vi "tip data FFT.vi"() -> ()   [LabVIEW 2016]
uses:
  <vilib>/Analysis/4window.llb/windowTd.ctl
  <userlib>/_OpenG.lib/array/array.llb/Sort 1D Array (DBL)__ogtk.vi
  <userlib>/_OpenG.lib/array/array.llb/Reorder 1D Array2 (DBL)__ogtk.vi
  <vilib>/measure/maresamp.llb/Resample Pair of Arrays (single shot).vi
  <vilib>/measure/maspectr.llb/FFT Power Spectrum and PSD for 1 Chan.vi
  <vilib>/measure/NI_MAPro.lvlib
  <vilib>/Analysis/NI_AALPro.lvlib
panel:
  in  "window":T1=3 items=["Rectangle"=0, "Hanning"=1, "Hamming"=2, "Blackman-Harris"=3, "Exact Blackman"=4, "Blackman"=5, "Flat Top"=6, "4 Term B-Harris "=7, "7 Term B-Harris"=8, "Low Sidelobe"=9, "Blackman Nuttall"=11, "Triangle"=30, "Bartlett-Hanning"=31, "Bohman"=32, "Parzen"=33, "Welch"=34, "Kaiser"=60, "Dolph-Chebyshev"=61, "Gaussian"=62]
  in  "t0":dbl=1.15 format="%.2p"
  in  "dt":dbl=1e-05 format="%.2p"
  out "Resampled data":waveform(dbl)(graph)={"t0"=timestamp(1.15 s since 1904-01-01), "dt"=1e-05, "Y"=[]}
  out "FFT (1/um)":cluster{"f0":dbl, "df":dbl, "magnitude":dbl[]}(graph)={"f0"=0.0, "df"=2.940052332931526, "magnitude"=[]}
  out "flattened superlattice":cluster{dbl[], dbl[]}(graph)
  in  "flatten superlattice angle":dbl=-34.65 format="%#_13g"
  in  "superlattice":cluster{dbl[], dbl[]}(graph)
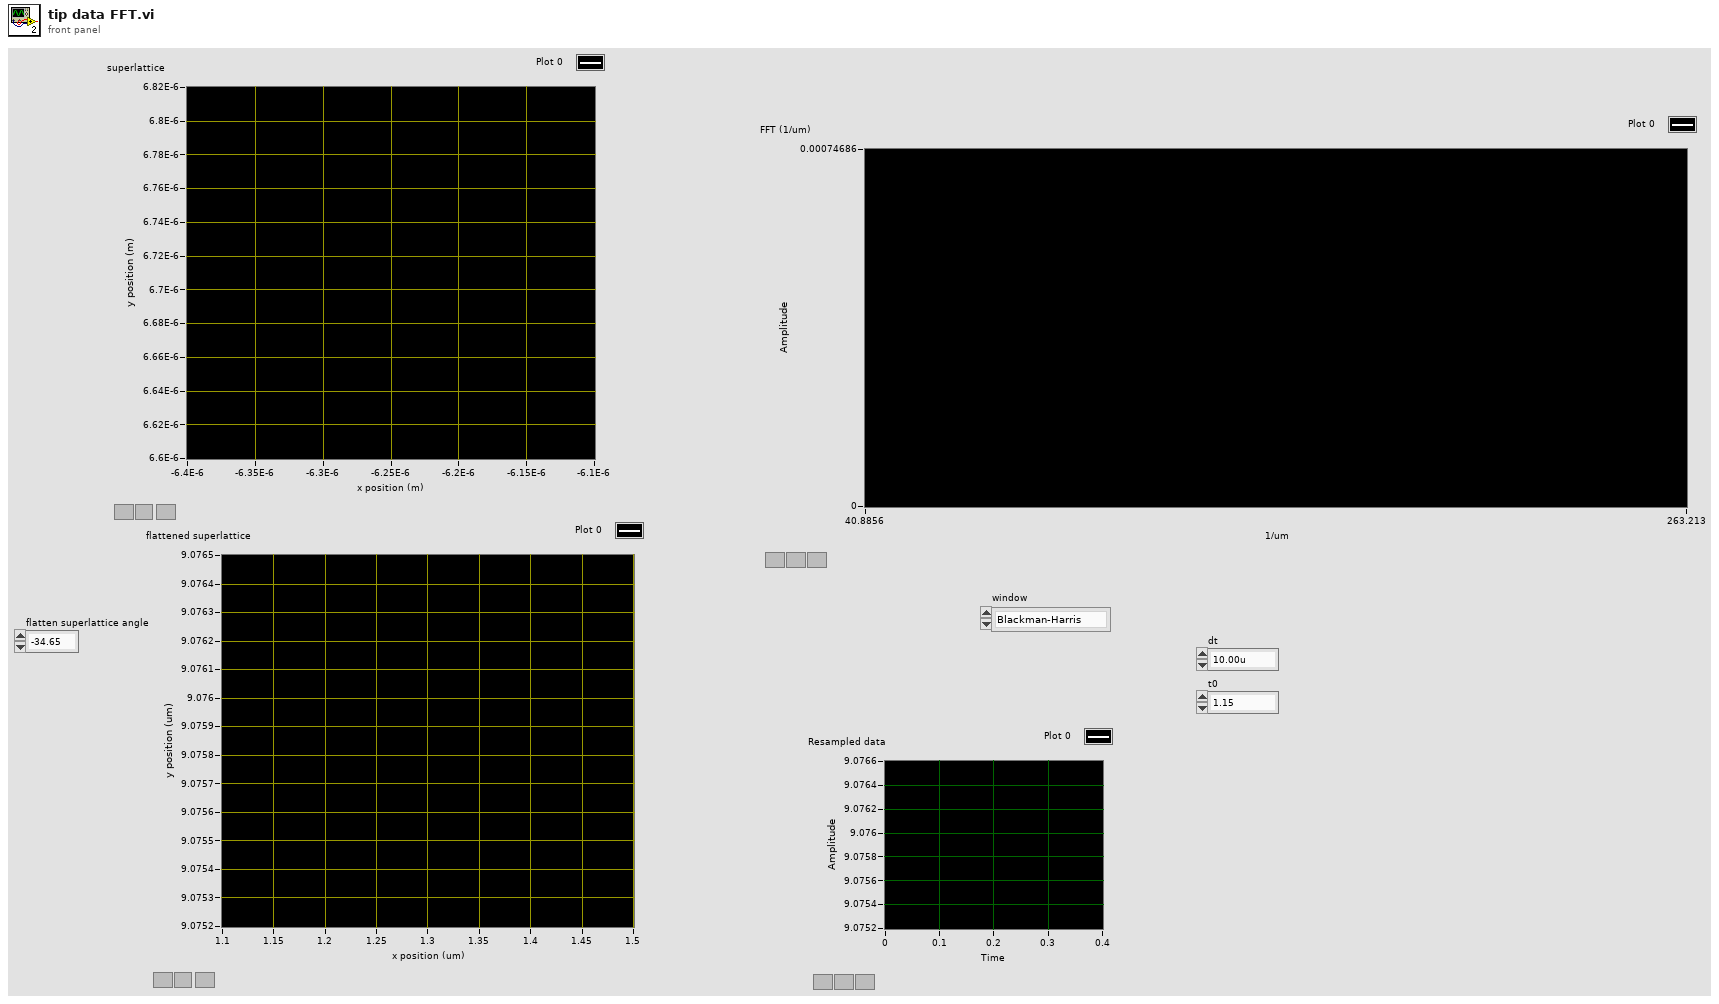
[diagram p1: front panel]
types:
  T1 = typedef "NI_AALPro.lvlib/windowTd.ctl" = u32
  T2 = cluster{"Sorted Array out":dbl[], "reordered array":dbl[]}
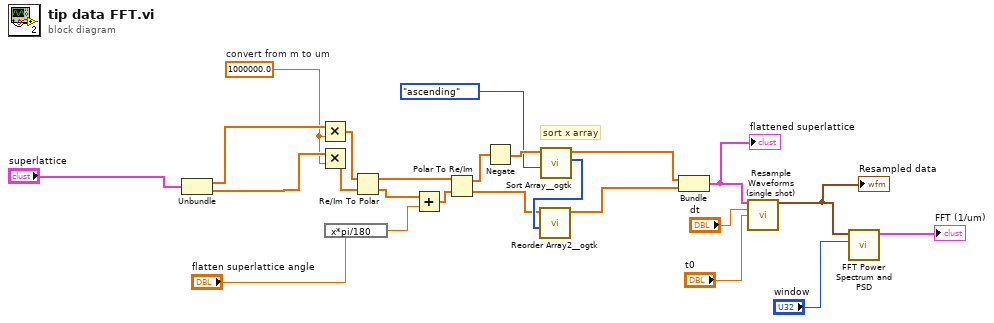
[diagram p0: block diagram]
diagram:
  w14 = 1000000.0  # convert from m to um
  # "sort x array"
  n1 = Unbundle("superlattice") -> (w16:dbl[], w15:dbl[])
  n2 = Multiply(x=w16, y=w14) -> (x*y=w12:dbl[])
  n3 = Multiply(x=w15, y=w14) -> (x*y=w13:dbl[])
  n4 = expression code="x*pi/180"("flatten superlattice angle") -> (w20:dbl)
  n5 = Re/Im To Polar(2:w13, 3:w12) -> (0:w24:dbl[], 1:w23:dbl[])
  n6 = Add(x=w24, y=w20) -> (x+y=w22:dbl[])
  n7 = Polar To Re/Im(2:w22, 3:w23) -> (0:w5:dbl[], 1:w9:dbl[])
  n8 = Negate(x=w9) -> (-x=w8:dbl[])
  n9 = call-poly <userlib>:"Sort Array__ogtk.vi"("Order"=enum16{"ascending", "descending"}."ascending", "Array in"=w8) -> ("Sorted Pointers"=w6:i32[], "Sorted Array out"=w3:dbl[])  [unwired: 8 in]
  n10 = call-poly <userlib>:"Reorder Array2__ogtk.vi"("indices"=w6, "array"=w5) -> ("reordered array"=w2:dbl[])  [unwired: 9 in]
  n11 = Bundle("Sorted Array out"=w3, "reordered array"=w2) -> (w11:T2)  [unwired: 1 in]
  "flattened superlattice" <- w11
  n12 = call-poly <vilib>:"Resample Waveforms (single shot).vi"("XY-data in"=w11, "dt"="dt", "t0"="t0") -> ("resampled waveform out"=w18:waveform(dbl))  [unwired: 8 in, 4 out]
  "Resampled data" <- w18
  n13 = call-poly <vilib>:"FFT Power Spectrum and PSD.vi"("window"="window", "time signal"=w18) -> ("Power Spectrum / PSD"=→"FFT (1/um)":cluster{"f0":dbl, "df":dbl, "magnitude":dbl[]})  [unwired: 6 in, 3 out]
